vi "publisher tests Writer 8.vi"() -> ()   [LabVIEW 2018]
uses:
  publisher action.ctl
panel:
  out "Numeric":i32
  out "number":dbl
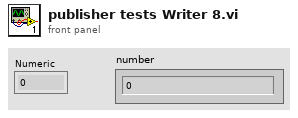
[diagram p1: front panel]
types:
  T1 = typedef "publisher action.ctl" = enum16{"set", "get", "init", "check"}
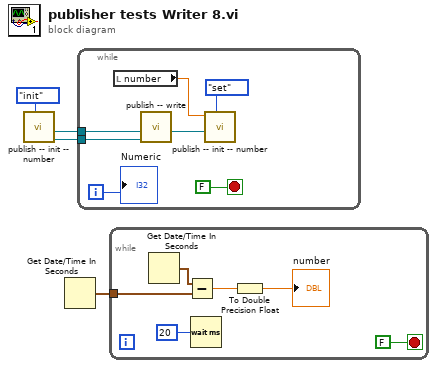
[diagram p0: block diagram]
diagram:
  n1 = call "publish -- init -- number.vi"("publisher action"=publisher_action."init") -> ("request event"=w2:refnum<user-event>, "recieve event"=w1:refnum<user-event>)  [unwired: 8 in, 1 out]
  n2 = Get Date/Time In Seconds() -> (seconds since 1Jan1904=w4:timestamp)
  n3 = while {
    tunnel: w2 -> [w9]
    tunnel: w1 -> [w8]
    i -> [w10]
    stop <- FALSE stop-if-true
    n4 = local read "number"() -> (w5:dbl)
    n5 = call "publish -- write.vi"("request event"=w9, "response event"=w8) -> ("response event OUT"=w7:refnum<user-event>)  [unwired: 9 in]
    n6 = call "publish -- init -- number.vi"("publisher action"=publisher_action."set", "recieve event IN"=w7, "Numeric"=w5) -> ()  [unwired: 6 in, 3 out]
    "Numeric" <- w10
  }
  n7 = while {
    tunnel: w4 -> [w14]
    stop <- FALSE stop-if-true
    n8 = Get Date/Time In Seconds() -> (seconds since 1Jan1904=w16:timestamp)
    n9 = Subtract(x=w16, y=w14) -> (x-y=w17:dbl)
    n10 = Wait (ms)(milliseconds to wait=u32 20) -> ()  [unwired: 1 out]
    n11 = To Double Precision Float(number=w17) -> (double precision float=→"number":dbl)
  }
